vi "PLC.Debug.Changeover.vi"(8 "error in (no error)":errorcluster, 10 "PLCchangeover":T2, 11 "Idx":i32) -> (0 "error out":errorcluster, 2 "PCchangeover":T1 {"TVH" format="%.3f"; "TVL" format="%.3f"; "TP" format="%.3f"})   [LabVIEW 2016]
doc: "Connect to PLC\n\nWabco 2017 All right reserved\nAuthor: maciej.szupienko@wabco-auto.com"
uses:
  LowLevel/PLC.DataBlock.PLCchangeover.ctl
  LowLevel/PLC.DataBlock.PCchangeover.ctl
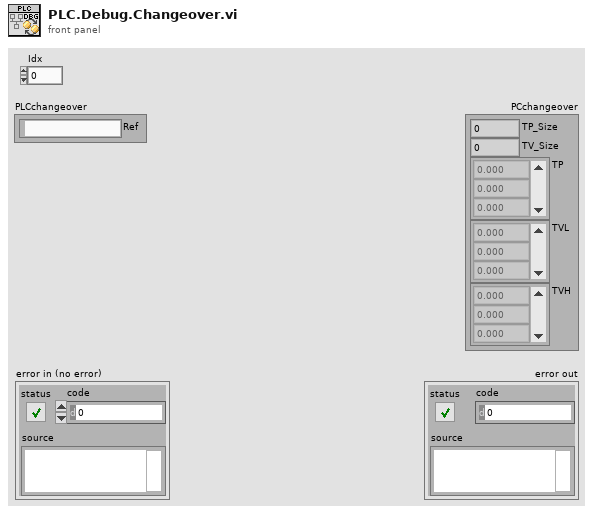
[diagram p1: front panel]
types:
  T1 = typedef "PLC.DataBlock.PCchangeover.ctl" = cluster{"TP_Size":u8, "TV_Size":u8, "TP":sgl[], "TVL":sgl[], "TVH":sgl[]}
  T2 = typedef "PLC.DataBlock.PLCchangeover.ctl" = cluster{"Ref":string}
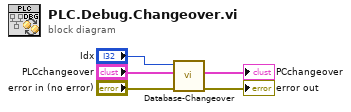
[diagram p0: block diagram]
diagram:
  n1 = call "Database-Changeover.vi"("error in"="error in (no error)", "PLCchangeover"="PLCchangeover", "Idx"="Idx") -> ("error out"=→"error out":errorcluster, "PCchangeover"=→"PCchangeover":T1)  [unwired: 7 in]
